vi "Trigger Analog Channel Read.vi"() -> ()   [LabVIEW 2020]
uses:
  <instrlib>/BDAQ-6104/Private/Edge Triger Type.ctl
  <instrlib>/BDAQ-6104/Public/Data/Read Single Analog Channel.vi
  <instrlib>/BDAQ-6104/BDAQ-6104.lvlib
panel:
  out "Trigger Activated":bool
  in  "Abort":bool
  out "Waveform Chart":dbl(graph)
  in  "Sample Period (ms)":u32=50
  in  "stop":bool
  in  "Channel":T1(ring)
  in  "VISA resource name":refnum<visa-resource-name>
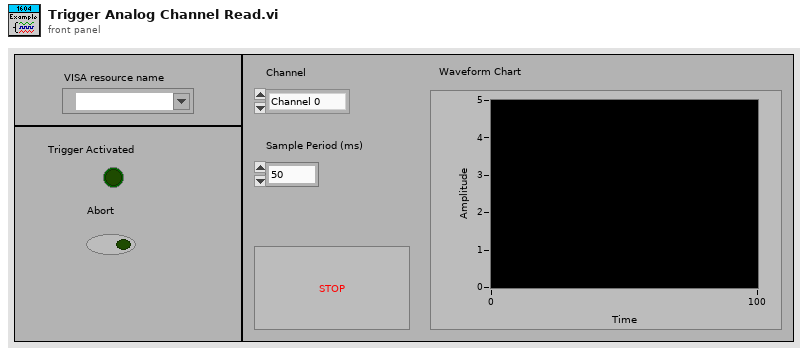
[diagram p1: front panel]
types:
  T1 = enum16{"Channel 0", "Channel 1", "Channel 2", "Channel 3", "Channel 4", "Channel 5"}
  T2 = typedef "BDAQ-6104.lvlib/Edge Triger Type.ctl" = enum16{"CHANGE", "FALLING", "RISING"}
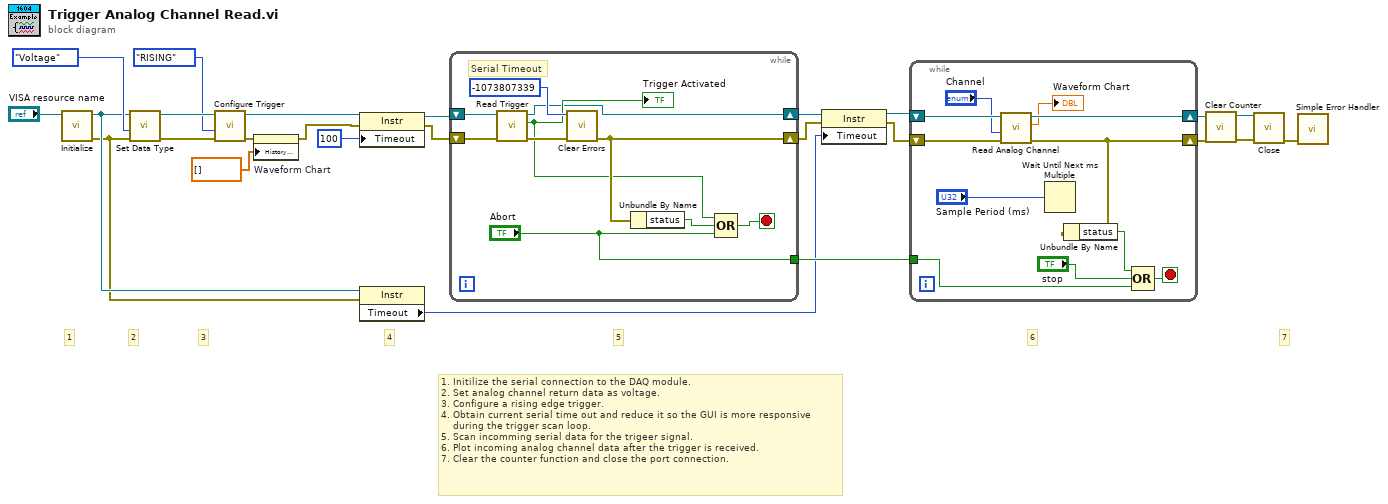
[diagram p0: block diagram]
diagram:
  # "1. Initilize the serial connection to the DAQ module.\n2. Set analog channel return data as voltage.\n3. Configure a rising edge trigger.\n4. Obtain current serial time out and reduce it so the GUI is more responsive \n    during the trigger scan loop.\n5. Scan incomming serial data for the trigeer signal.\n6. Plot incoming analog channel data after the trigger is received. \n7. Clear the counter function and close the port connection."
  # "7"
  # "6"
  # "5"
  # "4"
  # "3"
  # "2"
  # "1"
  n1 = call <instrlib>:"Initialize.vi"("VISA resource name"="VISA resource name") -> ("error out"=w16:errorcluster, "VISA resource name out"=w17:refnum<visa-resource-name>)  [unwired: 9 in]
  n2 = call <instrlib>:"Set Data Type.vi"("error in (no error)"=w16, "Data Type"=enum16{"Voltage", "Raw"}."Voltage", "VISA resource name"=w17) -> ("error out"=w3:errorcluster, "VISA resource name out"=w4:refnum<visa-resource-name>)  [unwired: 7 in]
  n3 = call <instrlib>:"Configure Trigger.vi"("error in (no error)"=w3, "Mode"=Edge_Triger_Type."RISING", "VISA resource name"=w4) -> ("error out"=w5:errorcluster, "VISA resource name out"=w2:refnum<visa-resource-name>)  [unwired: 7 in]
  n4 = property on="Waveform Chart" class="WFChart (strict)"(error in=w5, "History Data"=dbl[] []) -> (error out=w7:errorcluster)  [unwired: 1 in, 1 out]
  n5 = property class="Instr"(reference=w2, error in=w7, "Timeout"=u32 100 ("General Settings:Timeout Value")) -> (reference out=w14:refnum<visa-resource-name>, error out=w13:errorcluster)
  n6 = property class="Instr"(reference=w17, error in=w16) -> ("Timeout"=w8:u32)  [unwired: 2 out]
  n7 = while {
    shift-right: [w29] -> w11
    shift-left: w13 -> [w33]
    shift-right: [w27] -> w12
    shift-left: w14 -> [w32]
    tunnel: ["Abort"] -> w18
    stop <- w34 stop-if-true
    # "Serial Timeout"
    n8 = call <instrlib>:"Read Trigger.vi"("error in (no error)"=w33, "VISA resource name"=w32) -> ("error out"=w31:errorcluster, "Trigger Activated"=w28:bool, "VISA resource name out"=w27:refnum<visa-resource-name>)  [unwired: 7 in]
    "Trigger Activated" <- w28
    n9 = call <vilib>:"Clear Errors.vi"("error in (no error)"=w31, "specific error code to clear (0: all)"=-1073807339 ("y")) -> ("error out"=w29:errorcluster)  [unwired: 4 in, 1 out]
    n10 = Unbundle By Name(w29) -> ("status"=w35:bool)
    n11 = Compound Arithmetic op=OR(w28, w35, "Abort") -> (w34:bool)
  }
  n12 = property class="Instr"(reference=w12, error in=w11, "Timeout"=w8) -> (reference out=w9:refnum<visa-resource-name>, error out=w10:errorcluster)
  n13 = while {
    shift-right: [w45] -> w21
    shift-left: w9 -> [w46]
    shift-right: [w38] -> w20
    shift-left: w10 -> [w44]
    tunnel: w18 -> [w36]
    stop <- w37 stop-if-true
    n14 = call-poly <instrlib>:"Read Analog Channel.vi"("error in (no error)"=w44, "Channel"="Channel", "VISA resource name"=w46) -> ("error out"=w38:errorcluster, "Channel Data"=→"Waveform Chart":dbl, "VISA resource name"=w45:refnum<visa-resource-name>)  [unwired: 6 in]
    n15 = Wait Until Next ms Multiple(millisecond multiple="Sample Period (ms)") -> ()  [unwired: 1 out]
    n16 = Unbundle By Name(w38) -> ("status"=w39:bool)
    n17 = Compound Arithmetic op=OR(w39, "stop", w36) -> (w37:bool)
  }
  n18 = call <instrlib>:"Clear Counter.vi"("error in (no error)"=w20, "VISA resource name"=w21) -> ("error out"=w22:errorcluster, "VISA resource name out"=w23:refnum<visa-resource-name>)  [unwired: 8 in]
  n19 = call <instrlib>:"Close.vi"("error in (no error)"=w22, "VISA resource name"=w23) -> ("error out"=w24:errorcluster)  [unwired: 9 in]
  n20 = call <vilib>:"Simple Error Handler.vi"("error in (no error)"=w24) -> ()  [unwired: 4 in, 5 out]
